vi "pagessteps_rowspins_colssites.vi"() -> ()   [LabVIEW 2013]
panel:
  out "Array":dbl[][][](array[numeric]) format="%#_2g"
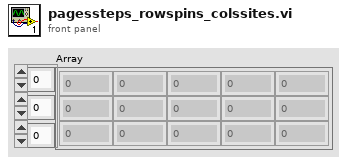
[diagram p1: front panel]
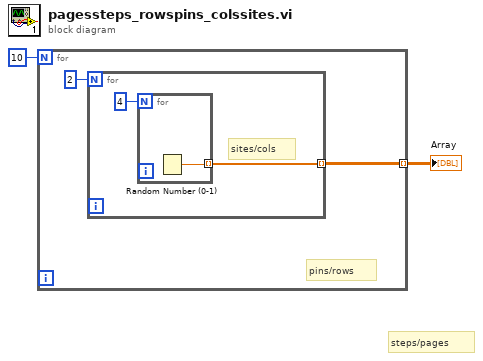
[diagram p0: block diagram]
diagram:
  # "steps/pages"
  n1 = for {
    N: 10 -> [_]
    tunnel: [w3] -> w1 mode=indexing
    # "pins/rows"
    n2 = for {
      N: 2 -> [_]
      tunnel: [w6] -> w3 mode=indexing
      # "sites/cols"
      n3 = for {
        N: 4 -> [_]
        tunnel: [w7] -> w6 mode=indexing
        n4 = Random Number (0-1)() -> (number: 0 to 1=w7:dbl)
      }
    }
  }
  "Array" <- w1
